vi "Chart Scale Count.vi"(8 "error in (no error)":errorcluster, 11 "Chart in":refnum<vi>) -> (0 "error out":errorcluster, 2 "Chart Scale Count":T1, 3 "Chart":refnum<vi>)   [LabVIEW 2020, in "VolatusGUIEditorCore.lvlib"]
uses:
  VolatusGUIEditorCore.lvlib
  Chart Scale Count.ctl
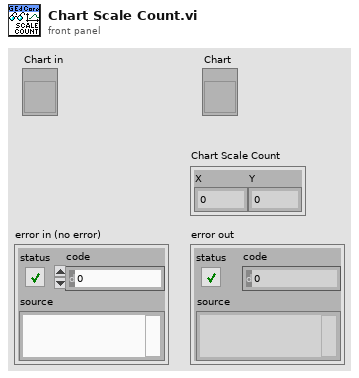
[diagram p1: front panel]
types:
  T1 = typedef "VolatusGUIEditorCore.lvlib/Chart Scale Count.ctl" = cluster{"X":i32, "Y":i32}
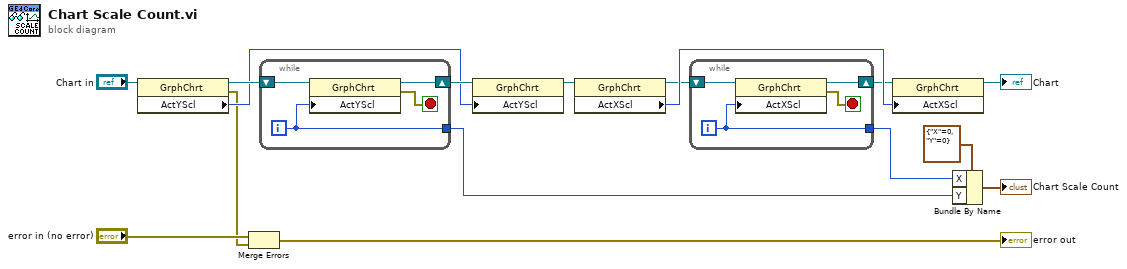
[diagram p0: block diagram]
diagram:
  n1 = property class="GrphChrt"(reference="Chart in") -> (reference out=w15:refnum<vi>, error out=w2:errorcluster, "ActYScl"=w13:i32)  [unwired: 1 in]
  n2 = Merge Errors("error in (no error)", w2) -> (→"error out":errorcluster)
  n3 = while {
    shift-right: [w18] -> w14
    shift-left: w15 -> [w20]
    tunnel: [w17] -> w4
    i -> [w17]
    stop <- w19 stop-if-true
    n4 = property class="GrphChrt"(reference=w20, "ActYScl"=w17) -> (reference out=w18:refnum<vi>, error out=w19:errorcluster)  [unwired: 1 in]
  }
  n5 = property class="GrphChrt"(reference=w14, "ActYScl"=w13) -> (reference out=w8:refnum<vi>)  [unwired: 1 in, 1 out]
  n6 = property class="GrphChrt"(reference=w8) -> (reference out=w10:refnum<vi>, "ActXScl"=w12:i32)  [unwired: 1 in, 1 out]
  n7 = while {
    shift-right: [w22] -> w11
    shift-left: w10 -> [w24]
    tunnel: [w21] -> w5
    i -> [w21]
    stop <- w23 stop-if-true
    n8 = property class="GrphChrt"(reference=w24, "ActXScl"=w21) -> (reference out=w22:refnum<vi>, error out=w23:errorcluster)  [unwired: 1 in]
  }
  n9 = property class="GrphChrt"(reference=w11, "ActXScl"=w12) -> (reference out=→"Chart":refnum<vi>)  [unwired: 1 in, 1 out]
  n10 = Bundle By Name(cluster=T1 {"X"=0, "Y"=0} ("Chart Scale Count"), "X"=w5, "Y"=w4) -> (→"Chart Scale Count":T1)
